vi "find_candidate_point.vi"(7 "Obstacle array":refnum<class "Obstacle.lvclass">[](array[class]), 9 "Distance from boat to waypoint":dbl, 10 "Candidate heading":dbl, 11 "Boat location":T1 {"North" format="%#_10f"; "East" format="%#_8f"}) -> (2 "Intermediate Point":T1 {"North" format="%#_10f"; "East" format="%#_8f"}, 3 "Point good?":bool)   [LabVIEW 2013]
doc: "This VI takes a boat location, a goal heading, the distance to the WP, and the obstacle array. It checks along the heading for twice as far as the distance from point to point and sees whether a point can be found that goes from point 1, to an intermediate point, to point 2.\n\nEric Schneider, September 2014"
uses:
  Data/TypeDefs/UTM Location.ctl
  Classes/Obstacle/Obstacle.lvclass
panel:
  in  "Number of loops to check":i32=20
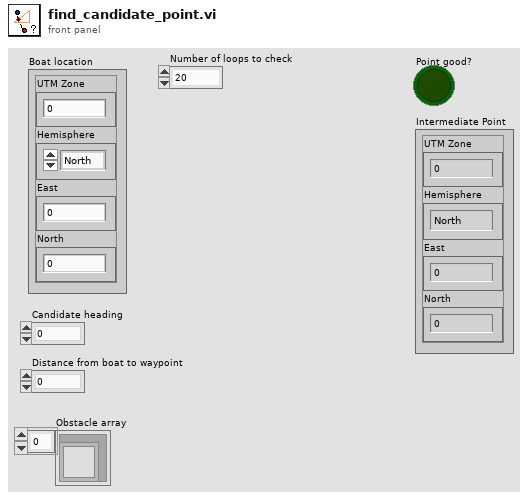
[diagram p1: front panel]
types:
  T1 = typedef "UTM Location.ctl" = cluster{"UTM Zone":dbl, "Hemisphere":enum16{"North", "South"}, "East":dbl, "North":dbl}
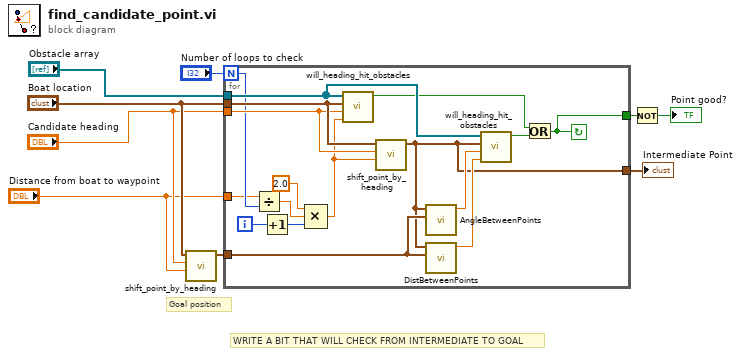
[diagram p0: block diagram]
diagram:
  # "Goal position"
  # "WRITE A BIT THAT WILL CHECK FROM INTERMEDIATE TO GOAL"
  n1 = call "shift_point_by_heading.vi"("Distance (m)"="Distance from boat to waypoint", "Heading (deg)"="Candidate heading", "UTM Point"="Boat location") -> ("Shifted UTM Point"=w4:T1)  [unwired: 8 in]
  n2 = for {
    N: "Number of loops to check" -> [w19]
    tunnel: "Boat location" -> [w25]
    tunnel: "Obstacle array" -> [w23]
    tunnel: "Candidate heading" -> [w24]
    tunnel: "Distance from boat to waypoint" -> [w18]
    tunnel: w4 -> [w15]
    tunnel: [w11] -> w3
    tunnel: [w10] -> w1
    i -> [w26]
    stop <- w11 continue-if-true
    n3 = Divide(x=w18, y=w19) -> (x/y=w17:dbl)
    n4 = Increment(x=w26) -> (x+1=w22:i32)
    n5 = Compound Arithmetic op=MULTIPLY(2.0 ("value"), w17, w22) -> (w20:dbl)
    n6 = call "will_heading_hit_obstacles.vi"("Distance to check (m)"=w20, "Heading"=w24, "Boat Location"=w25, "Obstacle array"=w23) -> ("Will boat hit any obstacles?"=w12:bool)  [unwired: 7 in]
    n7 = call "shift_point_by_heading.vi"("Distance (m)"=w20, "Heading (deg)"=w24, "UTM Point"=w25) -> ("Shifted UTM Point"=w10:T1)  [unwired: 8 in]
    n8 = call "AngleBetweenPoints.vi"("Point 2"=w15, "Point 1"=w10) -> ("Angle from P1 to P2"=w14:dbl)  [unwired: 9 in]
    n9 = call "DistBetweenPoints.vi"("UTM Location 2"=w15, "UTM Location 1"=w10) -> ("Distance from 1 to 2"=w16:dbl)  [unwired: 9 in]
    n10 = call "will_heading_hit_obstacles.vi"("Distance to check (m)"=w16, "Heading"=w14, "Boat Location"=w10, "Obstacle array"=w23) -> ("Will boat hit any obstacles?"=w13:bool)  [unwired: 7 in]
    n11 = Or(x=w12, y=w13) -> (x .or. y?=w11:bool)
  }
  "Intermediate Point" <- w1
  n12 = Not(x=w3) -> (.not. x?=→"Point good?":bool)
